vi "libssh2_agent_get_identity - invalid agent - end reached is TRUE.vi"() -> ()   [LabVIEW 2013, in "libssh2_tests.lvlib"]
uses:
  libssh2_tests.lvlib
  libssh2/Agent Refnum.ctl
  libssh2/libssh2_init_default.vi
  <vilib>/addons/_JKI Toolkits/Caraya/classes/Assert/Assert True.vi
  libssh2/libssh2.lvlib
  <vilib>/addons/_JKI Toolkits/Caraya/classes/Test/Test.lvclass
  <vilib>/addons/_JKI Toolkits/Caraya/classes/Assert/Assert.lvclass
panel:
  out "error out":errorcluster
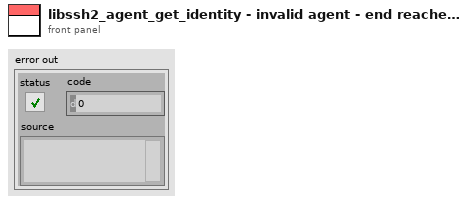
[diagram p1: front panel]
types:
  T1 = typedef "libssh2.lvlib/Agent Refnum.ctl" = refnum<k1>
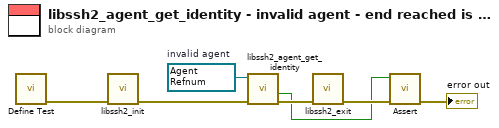
[diagram p0: block diagram]
diagram:
  w1 = T1 refnum items=["Agent"]  # invalid agent
  n1 = call <vilib>:"Define Test.vi"() -> ("error out"=w7:errorcluster)  [unwired: 10 in, 1 out]
  n2 = call-poly "libssh2_init.vi"("error in (no error)"=w7) -> ("error out"=w5:errorcluster)  [unwired: 10 in]
  n3 = call "libssh2_agent_get_identity.vi"("error in (no error)"=w5, "agent"=w1) -> ("error out"=w4:errorcluster, "end reached"=w2:bool)  [unwired: 7 in, 1 out]
  n4 = call "libssh2_exit.vi"("error in (no error)"=w4) -> ("error out"=w6:errorcluster)  [unwired: 10 in]
  n5 = call-poly <vilib>:"Assert.vi"("error in (no error)"=w6, "True?"=w2) -> ("error out"=→"error out":errorcluster)  [unwired: 8 in, 1 out]
